vi "FRCts20_Backend_Request_GET.vi"(6 "Message Attributes":T4, 8 "error in (no error)":errorcluster, 10 "Data":string, 11 "Engine_Refnums":T1) -> (0 "error out":errorcluster)   [LabVIEW 2013, in "FRCts20_Backend_Engine.lvlib"]
doc: "Returns a request's information and all notes from that request. Called by the Request API. Expects a request index"
uses:
  FRCts20_Backend_Engine.lvlib
  Dependencies/Keyed Array/KeyedArray.ctl
  FRCts20_Backend_EngineRefnums.ctl
  INI_Accessor/FRCts20_Backend_INI Controller.lvclass
  Dependencies/AMC/_SubVIs/TypeDefs/Message Queue.ctl
  Dependencies/AMC/_SubVIs/TypeDefs/Message.ctl
  <vilib>/addons/database/Connection.llb/Conn ObjectReference.ctl
  FRCts20_Backend_API/FRCts20_Backend_API_Request.ctl
  FRCts20_Backend_API/FRCts20_Backend_API_Status.ctl
  FRCts20_Backend_FGVOperation.ctl
  FRCts20_Backend_API/FRCts20_Backend_API.lvlib
  Dependencies/Keyed Array/Tools_KeyedArray.lvlib
  Dependencies/AMC/AMC.lvlib
  <vilib>/addons/database/NI_Database_API.lvlib
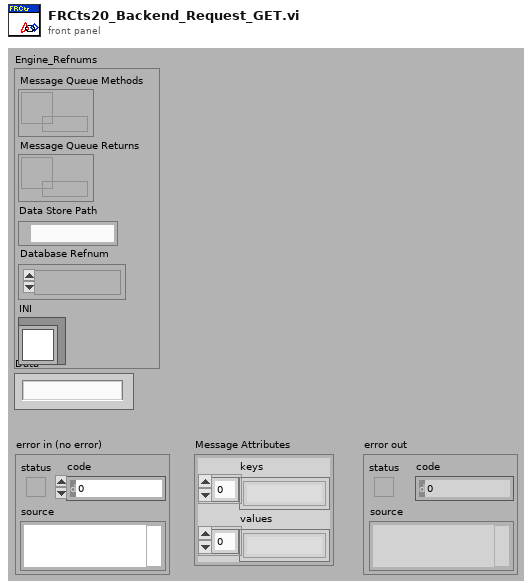
[diagram p1: front panel]
types:
  T1 = typedef "FRCts20_Backend_Engine.lvlib/FRCts20_Backend_EngineRefnums.ctl" = cluster{"Message Queue Methods":T2, "Message Queue Returns":T2, "Data Store Path":path, "Database Refnum":T3, "INI":refnum<class "FRCts20_Backend_INI Controller.lvclass">}
  T2 = typedef "AMC.lvlib/Message Queue.ctl" = refnum<queue>
  T3 = typedef "NI_Database_API.lvlib/Conn ObjectReference.ctl" = refnum<k1>
  T4 = typedef "Tools_KeyedArray.lvlib/KeyedArray.ctl" = cluster{"keys":string[], "values":string[]}
  T5 = typedef "FRCts20_Backend_Engine.lvlib/FRCts20_Backend_FGVOperation.ctl" = enum16{"Initialize", "EnqueueMessage", "EnqueueDataReturn", "FlushMessage", "FlushDataReturn"}
  T6 = typedef "FRCts20_Backend_API.lvlib/FRCts20_Backend_API_Request.ctl" = cluster{"Request Index":u32, "Description":string, "Status":T7, "Open Date":timestamp, "Last Update":timestamp, "Closed Date":timestamp, "Notes":cluster{"Note Index":u32, "Text":string, "Time Entered":timestamp, "Author":string, "Solution":bool}[], "Team Index":u32, "APIReturn":string}
  T7 = typedef "FRCts20_Backend_API.lvlib/FRCts20_Backend_API_Status.ctl" = enum16{"Open", "In Work", "Closed"}
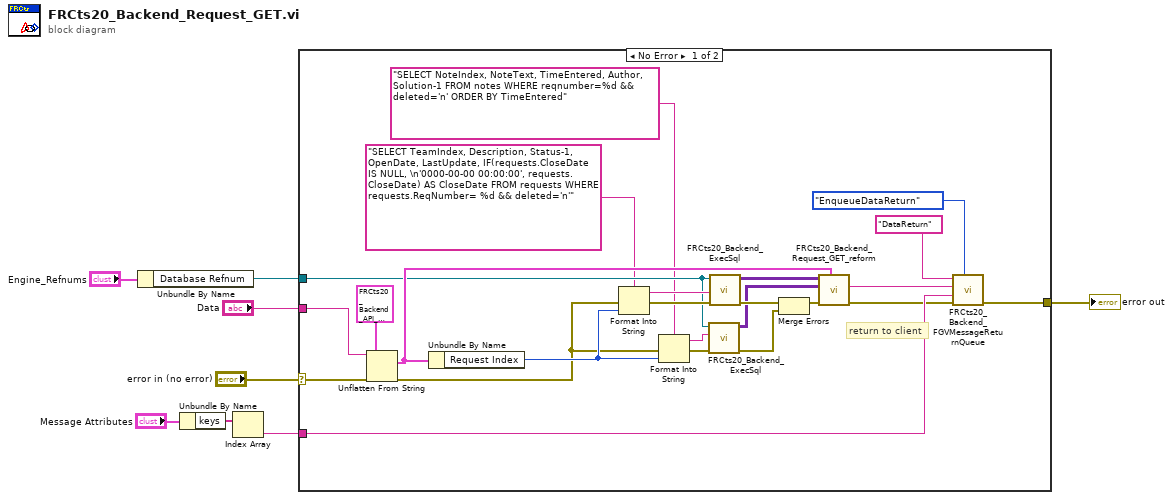
[diagram p0: block diagram]
diagram:
  n1 = Unbundle By Name("Engine_Refnums") -> ("Database Refnum"=w1:T3)
  n2 = Unbundle By Name("Message Attributes") -> ("keys"=w4:string[])
  n3 = Index Array(array=w4) -> (element=w3:string)  [unwired: 1 in]
  n4 = case shown="No Error" "error in (no error)" {
    selector: "error in (no error)" -> [w29 w33]
    tunnel: [w32 w33] -> w7
    tunnel: w1 -> [w15 _]
    tunnel: "Data" -> [w30 _]
    tunnel: w3 -> [w31 _]
    frame No Error {
      # "return to client"
      n5 = Unflatten From String(type=T6 {"Request Index"=0, "Description"="", "Status"=enum."Open", "Open Date"=timestamp(0 s since 1904-01-01), "Last Update"=timestamp(0 s since 1904-01-01), "Closed Date"=timestamp(0 s since 1904-01-01), "Notes"=[], "Team Index"=0, "APIReturn"=""} ("Request"), binary string=w30, error in (no error)=w29) -> (value=w19:T6, error out=w13:errorcluster)  [unwired: 2 in, 1 out]
      n6 = Unbundle By Name(w19) -> ("Request Index"=w14:u32)
      n7 = Format Into String(format string="SELECT TeamIndex, Description, Status-1, OpenDate, LastUpdate, IF(requests.CloseDate IS NULL, \n'0000-00-00 00:00:00', requests.CloseDate) AS CloseDate FROM requests WHERE requests.ReqNumber= %d && deleted='n'", error in=w13, w14) -> (resulting string=w23:string, error out=w22:errorcluster)  [unwired: 1 in]
      n8 = Format Into String(format string="SELECT NoteIndex, NoteText, TimeEntered, Author, Solution-1 FROM notes WHERE reqnumber=%d && deleted='n' ORDER BY TimeEntered", error in=w13, w14) -> (resulting string=w11:string, error out=w12:errorcluster)  [unwired: 1 in]
      n9 = call "FRCts20_Backend_ExecSql.vi"("error in (no error)"=w12, "format string"=w11, "Refnum in"=w15) -> ("error out"=w16:errorcluster, "recordset data"=w18:variant[][])  [unwired: 6 in, 1 out]
      n10 = call "FRCts20_Backend_ExecSql.vi"("error in (no error)"=w22, "format string"=w23, "Refnum in"=w15) -> ("error out"=w20:errorcluster, "recordset data"=w21:variant[][])  [unwired: 6 in, 1 out]
      n11 = Merge Errors(w20, w16) -> (w17:errorcluster)
      n12 = call "FRCts20_Backend_Request_GET_reform.vi"("Request"=w19, "error in (no error)"=w17, "note data"=w18, "request data"=w21) -> ("error out"=w26:errorcluster, "data string"=w27:string)  [unwired: 6 in]
      n13 = call "FRCts20_Backend_FGVMessageReturnQueue.vi"("Operation"=FRCts20_Backend_FGVOperation."EnqueueDataReturn", "error in (no error)"=w26, "Key"=w31, "Message Value"=w27, "Message Name"="DataReturn") -> ("error out"=w32:errorcluster)  [unwired: 5 in, 1 out]
    }
    frame Error {
    }
  }
  "error out" <- w7
